vi "Destroy.vi"(8 "error in (no error)":errorcluster, 11 "CSM-Helper in":refnum<class "CSM-Helper.lvclass">) -> (0 "error out":errorcluster, 3 "CSM-Helper out":refnum<class "CSM-Helper.lvclass">)   [LabVIEW 2020, in "CSM-Helper.lvclass"]
uses:
  CSM-Helper.lvclass
  CSM-Helper.lvclass/CSM-Helper.ctl
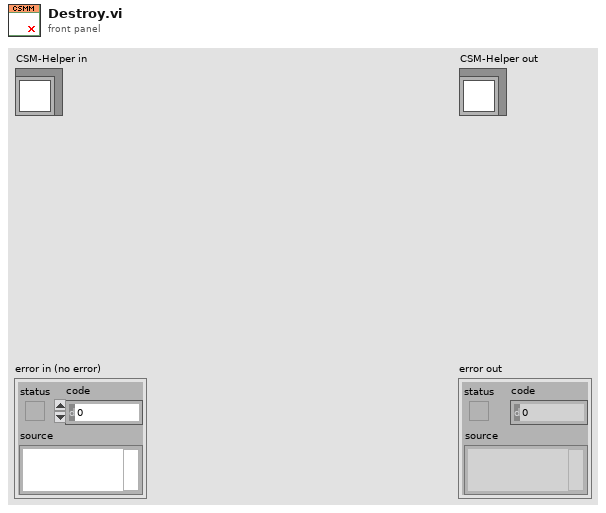
[diagram p1: front panel]
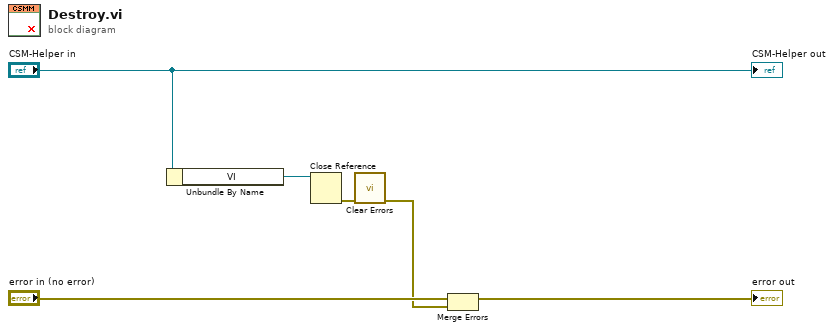
[diagram p0: block diagram]
diagram:
  n1 = Unbundle By Name("CSM-Helper in") -> ("VI"=w4:refnum<vi>)
  n2 = Close Reference(reference=w4) -> (error out=w3:errorcluster)  [unwired: 1 in]
  n3 = call <vilib>:"Clear Errors.vi"("error in (no error)"=w3) -> ("error out"=w1:errorcluster)  [unwired: 5 in, 1 out]
  n4 = Merge Errors("error in (no error)", w1) -> (→"error out":errorcluster)
  "CSM-Helper out" <- "CSM-Helper in"
